vi "elapsed time with FGV.vi"(8 "error in (no error)":errorcluster) -> (0 "error out":errorcluster, 2 "elapsed time, s":dbl)   [LabVIEW 2018, in "LabView-0mq-Jl_Roundtrip_lib.lvlib"]
uses:
  LabView-0mq-Jl_Roundtrip_lib.lvlib
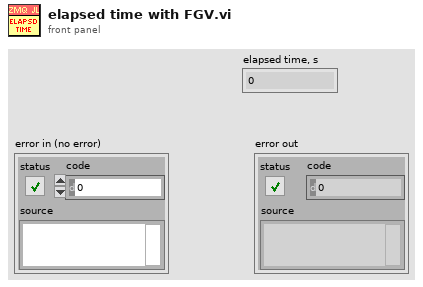
[diagram p1: front panel]
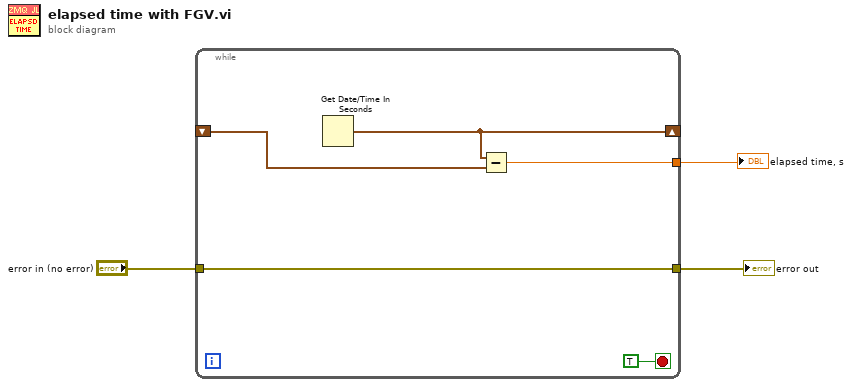
[diagram p0: block diagram]
diagram:
  n1 = while {
    tunnel: [w7] -> w3
    tunnel: "error in (no error)" -> [w7]
    shift-right: [w6] -> _
    shift-left: _ -> [w5]
    tunnel: [w4] -> w1
    stop <- TRUE stop-if-true
    n2 = Get Date/Time In Seconds() -> (seconds since 1Jan1904=w6:timestamp)
    n3 = Subtract(x=w6, y=w5) -> (x-y=w4:dbl)
  }
  "elapsed time, s" <- w1
  "error out" <- w3
